vi "Do.vi"(8 "error in":errorcluster, 10 "Actor in":refnum<class "Actor.lvclass">, 11 "Update TEC Multipliers":refnum<class "Update TEC Multipliers.lvclass">) -> (0 "error out":errorcluster, 2 "Actor out":refnum<class "Actor.lvclass">)   [LabVIEW 2014, in "TE Cooler.lvlib" / "Update TEC Multipliers.lvclass"]
doc: "(<B>Filename</B>: Actor Framework.lvlib:Message.lvclass:Do.vi)\n\nDefines what a message does when it is received by an actor. Generally, a message instructs an actor to invoke one of its methods. By default, this method does nothing. A child class must override it to define behavior. Create a child class by using the Actor Framework Message Maker dialog box."
uses:
  Update TEC Multipliers.lvclass
  <vilib>/ActorFramework/Actor/Actor.lvclass
  Update TEC Multipliers.lvclass/Update TEC Multipliers.ctl
  reusable/DAQ Device/Device/Device.lvclass
  reusable/DAQ Device/Device/Device.lvclass/Device.ctl
  SuperActor/SuperActor.lvclass/SuperActor.ctl
  Devices/TE Cooler/TE Cooler.lvclass
  reusable/DAQ Device/Device/Read Configurable Device.vi
  SuperActor/Read ID.vi
  SuperActor/Read Log Session.vi
  SuperActor/Read CVT Session.vi
  Devices/TE Cooler/Write Cool Side Multiplier.vi
  Devices/TE Cooler/Write Heat Side Multiplier.vi
  <userlib>/_Session Fwk/Session - Root.lvclass
  Devices/Configurable Device/Configurable Device.lvclass
  reusable/Session APIs/CVT/CVT.lvclass
  reusable/Session APIs/Session Log/System Log.lvclass
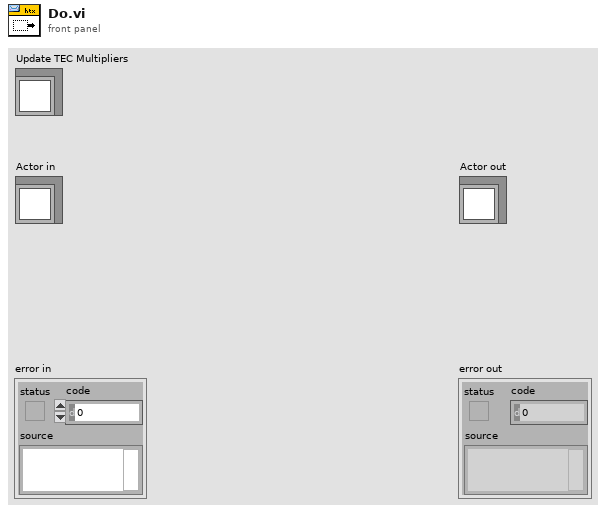
[diagram p1: front panel]
types:
  T1 = typedef "Session - Root.lvclass/Session Handle.ctl" = refnum<data-value>
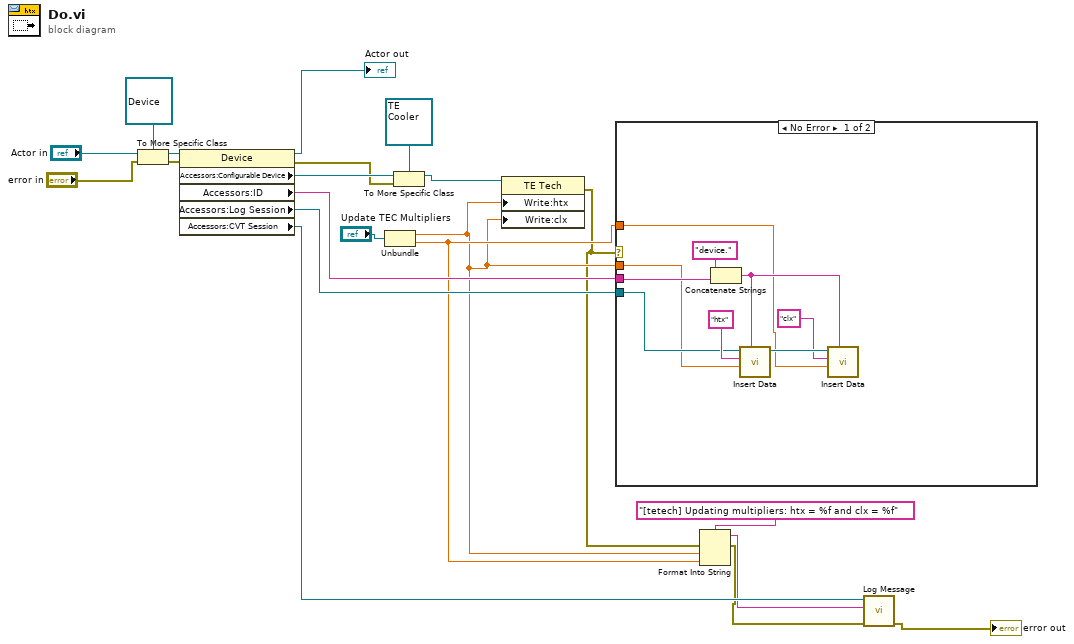
[diagram p0: block diagram]
diagram:
  n1 = To More Specific Class(target class=refnum<class "Device.lvclass"> refnum ("DAQ Device.lvlib:Device"), reference="Actor in", error in="error in") -> (specific class reference=w19:refnum<class "Device.lvclass">, error out=w14:errorcluster)
  n2 = property class="Device"(reference=w19, error in=w14) -> (reference out=→"Actor out":refnum<class "Device.lvclass">, error out=w16:errorcluster, "Accessors:Configurable Device"=w18:refnum<class "Configurable Device.lvclass">, "Accessors:ID"=w11:string, "Accessors:Log Session"=w12:T1, "Accessors:CVT Session"=w10:T1)
  n3 = Unbundle("Update TEC Multipliers") -> (w2:dbl, w4:dbl)
  n4 = To More Specific Class(target class=refnum<class "TE Cooler.lvclass"> refnum ("TE Cooler.lvlib:TE Tech"), reference=w18, error in=w16) -> (specific class reference=w3:refnum<class "TE Cooler.lvclass">)  [unwired: 1 out]
  n5 = property class="TE Tech"(reference=w3, "Write:htx"=w2, "Write:clx"=w2) -> (error out=w1:errorcluster)  [unwired: 1 in, 1 out]
  n6 = case shown="No Error" w1 {
    tunnel: w12 -> [w27 _]
    tunnel: w11 -> [w28 _]
    tunnel: w2 -> [w23 _]
    tunnel: w4 -> [w22 _]
    frame No Error {
      n7 = Concatenate Strings("device." ("string"), w28) -> (w24:string)
      n8 = call "Insert Data.vi"("Group"=w24, "Data"=w23, "tag"="htx", "CVT Session In"=w27) -> ("CVT Session Out"=w26:T1)  [unwired: 6 in, 1 out]
      n9 = call "Insert Data.vi"("Group"=w24, "Data"=w22, "tag"="clx", "CVT Session In"=w26) -> ()  [unwired: 6 in, 2 out]
    }
    frame Error {
    }
  }
  n10 = Format Into String(format string="[tetech] Updating multipliers: htx = %f and clx = %f", error in=w1, w2, w4) -> (resulting string=w8:string, error out=w5:errorcluster)  [unwired: 1 in]
  n11 = call "Log Message.vi"("error in"=w5, "MSG In"=w8, "session in"=w10) -> ("error out"=→"error out":errorcluster)  [unwired: 7 in, 1 out]
